vi "Read input tags.vi"(8 "error in":errorcluster, 11 "current tag file io module runtime in":refnum<class "current tag file io module runtime.lvclass">=refnum) -> (0 "error out":errorcluster, 2 "input tags":T1[](array[typedef]), 3 "current tag file io module runtime out":refnum<class "current tag file io module runtime.lvclass">)   [LabVIEW 2013]
doc: "Copyright 2016 National Instruments Corporation\n\nLicensed under the Apache License, Version 2.0 (the \"License\"); you may not use this file except in compliance with the License. You may obtain a copy of the License at http://www.apache.org/licenses/LICENSE-2.0\nUnless required by applicable law or agreed to in writing, software distributed under the License is distributed on an \"AS IS\" BASIS, WITHOUT WARRANTIES OR CONDITIONS OF ANY KIND, either express or implied. See the License for the specific language governing permissions and limitations under the License."
uses:
  current tag file io module runtime.lvclass
  <vilib>/NI/Tag Bus/tag/Data Type.ctl
  <vilib>/NI/Tag Bus/tag/tag descriptor.lvclass
  current tag file io configuration.ctl
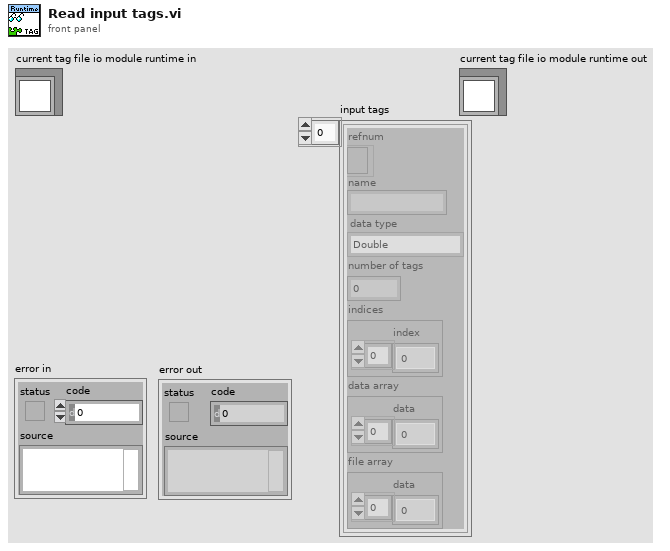
[diagram p1: front panel]
types:
  T1 = typedef "current tag file io module runtime.lvclass/current tag file io configuration.ctl" = cluster{"refnum":refnum<file>, "name":string, "data type":T2, "number of tags":i32, "indices":cluster{"index":i32[]}, "data array":cluster{"data":dbl[]}, "file array":cluster{"data":dbl[]}}
  T2 = typedef "tag bus.lvlib/tag descriptor.lvclass/Data Type.ctl" = enum16{"Double", "Single", "I64", "I32", "I16", "I8", "U64", "U32", "U16", "U8", "Boolean", "String", "Array of Double", "Array of Single", "Array of I64", "Array of I32", "Array of I16", "Array of I8", "Array of U64", "Array of U32", "Array of U16", "Array of U8", "Array of Boolean", "Array of String"}
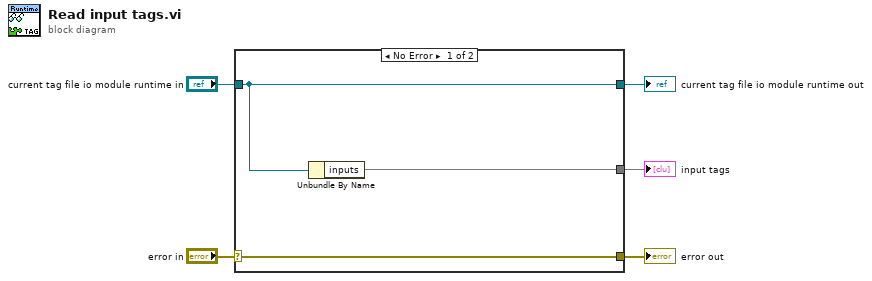
[diagram p0: block diagram]
diagram:
  n1 = case shown="No Error" "error in" {
    selector: "error in" -> [w8 w9]
    tunnel: [w8 w9] -> w4
    tunnel: [w7 w10] -> w2
    tunnel: "current tag file io module runtime in" -> [w7 w10]
    tunnel: [w6 _] -> w1
    frame No Error {
      n2 = Unbundle By Name(w7) -> ("inputs"=w6)
    }
    frame Error {
    }
  }
  "error out" <- w4
  "current tag file io module runtime out" <- w2
  "input tags" <- w1
